vi "Add Relay Channel.vi"(8 "error in (no error)":errorcluster, 10 "Relay Channel Data":T2, 11 "MUX Section Ref in":T1 format="%.0x") -> (0 "error out":errorcluster, 3 "MUX Section Ref out":T1 format="%.0x")   [LabVIEW 2013, in "MUX Custom Device.lvlib"]
uses:
  MUX Custom Device.lvlib
  <vilib>/NI Veristand/Custom Device API/Custom Device Item Ref.ctl
  Relay Channel Data.ctl
  Relay Data.ctl
  Switch.ctl
  <vilib>/NI Veristand/Custom Device API/Custom Device Channel.ctl
  <vilib>/NI Veristand/Custom Device API/Custom Device Channel Type.ctl
  MUX Global.vi
  <vilib>/NI Veristand/Custom Device API/Custom Device API.lvlib
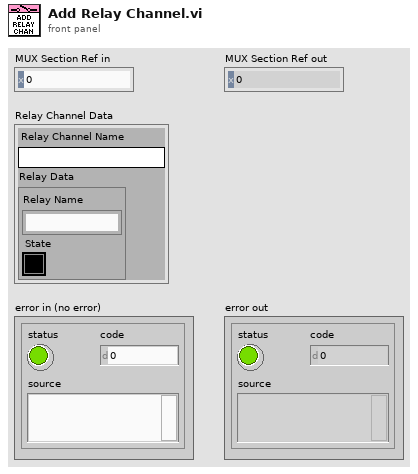
[diagram p1: front panel]
types:
  T1 = typedef "Custom Device API.lvlib/Custom Device Item Ref.ctl" = u64
  T2 = typedef "MUX Custom Device.lvlib/Relay Channel Data.ctl" = cluster{"Relay Channel Name":string, "Relay Data":T3}
  T3 = typedef "MUX Custom Device.lvlib/Relay Data.ctl" = cluster{"Relay Name":string, "State":T4}
  T4 = typedef "MUX Custom Device.lvlib/Switch.ctl" = bool
  T5 = typedef "Custom Device API.lvlib/Custom Device Channel.ctl" = cluster{"Type":T6, "Units":string, "Default Value":dbl, "Faultable":bool, "Scalable":bool}
  T6 = typedef "Custom Device API.lvlib/Custom Device Channel Type.ctl" = enum16{"Input", "Output"}
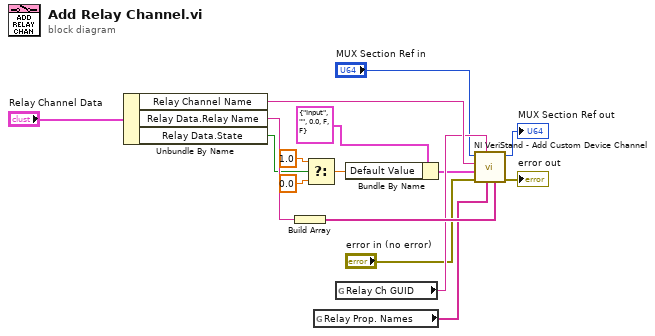
[diagram p0: block diagram]
diagram:
  n1 = Unbundle By Name("Relay Channel Data") -> ("Relay Channel Name"=w15:string, "Relay Data.Relay Name"=w16:string, "Relay Data.State"=w5:T4)
  n2 = Build Array(w16) -> (w14:string[])
  n3 = Select(t=1.0, s=w5, f=0.0) -> (s? t:f=w11:dbl)
  n4 = global read "MUX Global.vi" "Relay Prop. Names"() -> (w4:string[])
  n5 = global read "MUX Global.vi" "Relay Ch GUID"() -> (w13:string)
  n6 = Bundle By Name(cluster=T5 {"Type"=enum."Input", "Units"="", "Default Value"=0.0, "Faultable"=FALSE, "Scalable"=FALSE} ("Channel"), "Default Value"=w11) -> (w12:T5)
  n7 = call <vilib>:"NI VeriStand - Add Custom Device Channel.vi"("Property Values"=w14, "Property names"=w4, "GUID (Default Channel)"=w13, "error in (no error)"="error in (no error)", "Channel"=w12, "Channel Name"=w15, "Parent Ref in"="MUX Section Ref in") -> ("error out"=→"error out":errorcluster, "Parent Ref out"=→"MUX Section Ref out":T1)  [unwired: 1 in, 2 out]
